vi "Merge errors.vi"(9 "error in":errorcluster, 10 "Error to add":errorcluster) -> (3 "error out":errorcluster)   [LabVIEW 2020]
uses:
  WAMP Client/WAMP Client.lvclass/WAMP Client.ctl
  Utils.lvclass/Utils.ctl
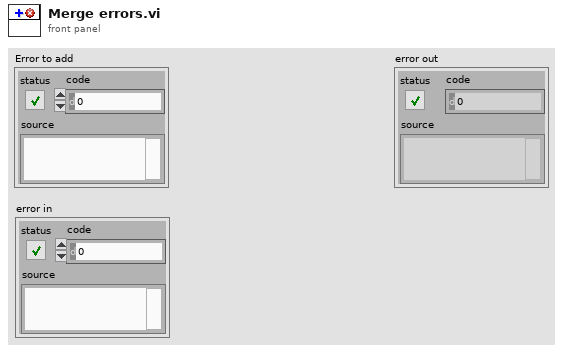
[diagram p1: front panel]
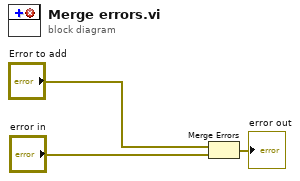
[diagram p0: block diagram]
diagram:
  n1 = Merge Errors("Error to add", "error in") -> (→"error out":errorcluster)
